vi "Close Connection--SubVI.vi"(8 "error in (no error)":errorcluster, 11 "Watlow F4T in":refnum<class "Watlow F4T.lvclass">) -> (0 "error out":errorcluster, 3 "Watlow F4T out":refnum<class "Watlow F4T.lvclass">)   [LabVIEW 2024, in "Watlow F4T.lvclass"]
uses:
  Watlow F4T.lvclass
  Watlow F4T.lvclass/Watlow F4T.ctl
  <instrlib>/Watlow Std Bus/Public/Watbus.dll
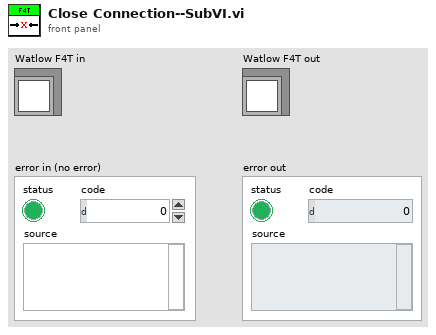
[diagram p1: front panel]
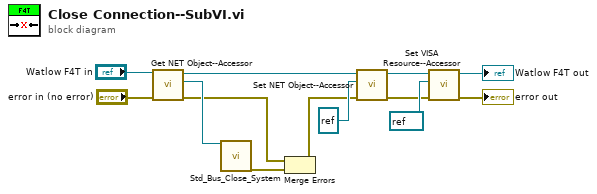
[diagram p0: block diagram]
diagram:
  n1 = call "Get NET Object--Accessor.vi"("error in (no error)"="error in (no error)", "Watlow F4T in"="Watlow F4T in") -> ("error out"=w9:errorcluster, ".NET Object"=w10:refnum<k24>, "Watlow F4T out"=w6:refnum<class "Watlow F4T.lvclass">)  [unwired: 7 in]
  n2 = call <instrlib>:"Std_Bus_Close_System.vi"("ILabVIEW In"=w10) -> ("error out"=w13:errorcluster)  [unwired: 18 in]
  n3 = Merge Errors(w9, w13) -> (w7:errorcluster)
  n4 = call "Set NET Object--Accessor.vi"("error in (no error)"=w7, ".NET Object"=refnum<k24> refnum, "Watlow F4T in"=w6) -> ("error out"=w4:errorcluster, "Watlow F4T out"=w3:refnum<class "Watlow F4T.lvclass">)  [unwired: 7 in]
  n5 = call-dynamic "Set VISA Resource--Accessor.vi"("error in (no error)"=w4, "VISA Resource"=refnum<visa-resource-name> refnum, "Watlow F4T in"=w3) -> ("error out"=→"error out":errorcluster, "Watlow F4T out"=→"Watlow F4T out":refnum<class "Watlow F4T.lvclass">)  [unwired: 7 in]
